vi "TempConversionSubVIMarcoGonzalez.vi"(2 "Boolean":bool, 3 "Temp":dbl) -> (1 "Converted Temp":dbl)   [LabVIEW 2012]
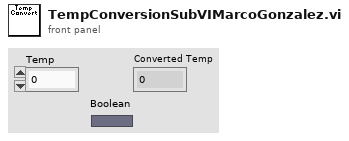
[diagram p1: front panel]
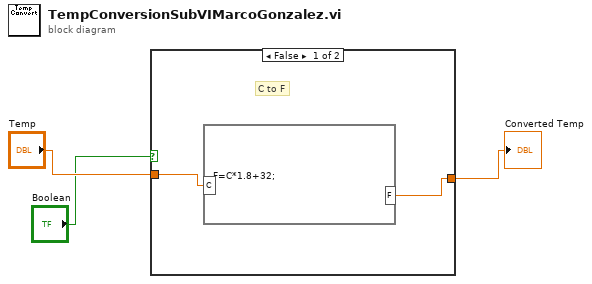
[diagram p0: block diagram]
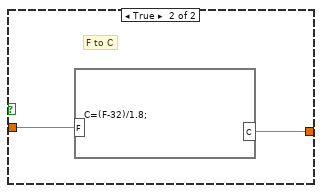
[diagram p2: hidden frame]
diagram:
  n1 = case shown="False" "Boolean" {
    tunnel: "Temp" -> [w4 w7]
    tunnel: [w5 w6] -> w1
    frame False {
      # "C to F"
      n2 = formula code="F=C*1.8+32;"("C"=w4) -> ("F"=w5:dbl)
    }
    frame True {
      # "F to C"
      n3 = formula code="C=(F-32)/1.8;"("F"=w7) -> ("C"=w6:dbl)
    }
  }
  "Converted Temp" <- w1
